vi "Score Particles2.vi"(6 "error in (no error)":errorcluster, 8 "Area Size Limit":i32=444, 9 "Particle Count Limit":i32=10, 11 "Image Refnum in":T1) -> (0 "error out":errorcluster, 2 "Scored Particle Info":T2(array[cluster]), 3 "Image Refnum out":T1)   [LabVIEW 2011]
doc: "Score the largest particles in the image to determine how well they match the target attributes. Specifically, calculate how rectangular a particle is, inspect its aspect ratio, and determine if it is hollow (having pixels on around the edges, but off in the large center)."
uses:
  <vilib>/vision/Image Controls.llb/IMAQ Image.ctl
  <vilib>/vision/NI_Vision_Development_Module.lvlib
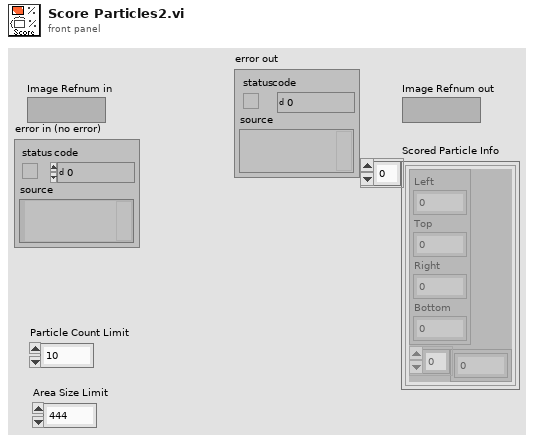
[diagram p1: front panel]
types:
  T1 = typedef "IMAQ Image.ctl" = refnum<image>
  T2 = cluster{cluster{"Left":dbl, "Top":dbl, "Right":dbl, "Bottom":dbl}, dbl[]}[]
  T3 = typedef "Particle Parameters" = i32
  T4 = typedef "Image Type" = u32
  T5 = cluster{"Left":dbl, "Top":dbl, "Right":dbl, "Bottom":dbl}
  T6 = cluster{cluster{"Left":dbl, "Top":dbl, "Right":dbl, "Bottom":dbl}, dbl[]}
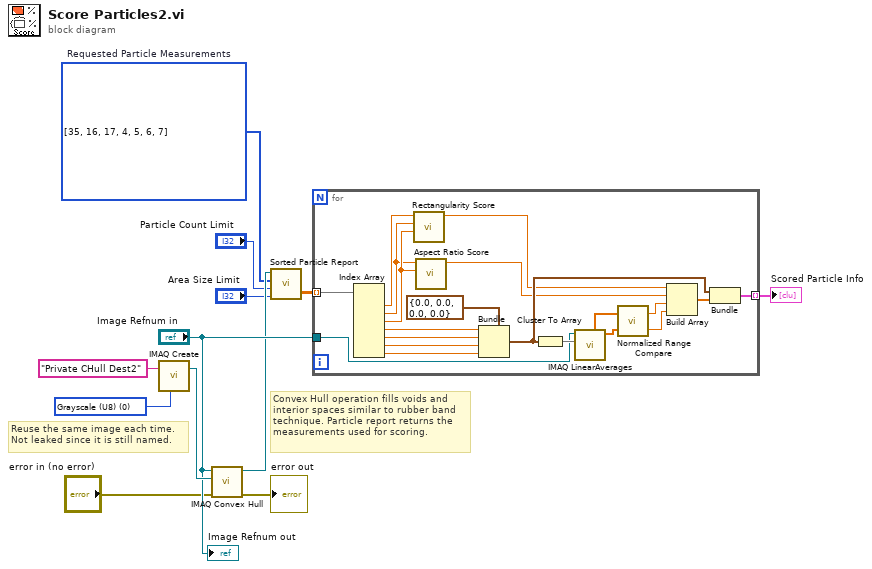
[diagram p0: block diagram]
diagram:
  w3 = T3[] [35, 16, 17, 4, 5, 6, 7] items=["Center of Mass X", "Center of Mass Y", "First Pixel X", "First Pixel Y", "Bounding Rect Left", "Bounding Rect Top", "Bounding Rect Right", "Bounding Rect Bottom", "Max Feret Diameter Start X", "Max Feret Diameter Start Y", "Max Feret Diameter End X", "Max Feret Diameter End Y", "Max Horiz. Segment Length Left", "Max Horiz. Segment Length Right", "Max Horiz. Segment Length Row", "-", "Bounding Rect Width", "Bounding Rect Height", "Bounding Rect Diagonal", "Perimeter", "Convex Hull Perimeter", "Holes' Perimeter", "Max Feret Diameter", "Equivalent Ellipse Major Axis", "Equivalent Ellipse Minor Axis", "Equivalent Ellipse Minor Axis (Feret)", "Equivalent Rect Long Side", "Equivalent Rect Short Side", "Equivalent Rect Diagonal", "Equivalent Rect Short Side (Feret)", "Average Horiz. Segment Length", "Average Vert. Segment Length", "Hydraulic Radius", "Waddel Disk Diameter", "-", "Area", "Holes' Area", "Particle & Holes' Area", "Convex Hull Area", "Image Area", "-", "Number of Holes", "Number of Horiz. Segments", "Number of Vert. Segments", "-", "Orientation", "Max Feret Diameter Orientation", "-", "% Area/Image Area", "% Area/(Particle & Holes' Area)", "Ratio of Equivalent Ellipse Axes", "Ratio of Equivalent Rect Sides", "-", "Elongation Factor", "Compactness Factor", "Heywood Circularity Factor", "Type Factor", "-", "Sum X", "Sum Y", "Sum XX", "Sum XY", "Sum YY", "Sum XXX", "Sum XXY", "Sum XYY", "Sum YYY", "-", "Moment of Inertia XX", "Moment of Inertia XY", "Moment of Inertia YY", "Moment of Inertia XXX", "Moment of Inertia XXY", "Moment of Inertia XYY", "Moment of Inertia YYY", "Norm. Moment of Inertia XX", "Norm. Moment of Inertia XY", "Norm. Moment of Inertia YY", "Norm. Moment of Inertia XXX", "Norm. Moment of Inertia XXY", "Norm. Moment of Inertia XYY", "Norm. Moment of Inertia YYY", "Hu Moment 1", "Hu Moment 2", "Hu Moment 3", "Hu Moment 4", "Hu Moment 5", "Hu Moment 6", "Hu Moment 7"]  # Requested Particle Measurements
  w9 = T4 0 items=["Grayscale (U8)", "Grayscale (I16)", "Grayscale (SGL)", "Complex (CSG)", "RGB (U32)", "HSL (U32)", "RGB (U64)", "Grayscale (U16)"] ("Image Type")
  # "Reuse the same image each time.\nNot leaked since it is still named."
  # "Convex Hull operation fills voids and\ninterior spaces similar to rubber band\ntechnique. Particle report returns the\nmeasurements used for scoring."
  n1 = call "IMAQ Create"("Image Name"="Private CHull Dest2", "Image Type"=w9) -> ("New Image"=w8:T1)  [unwired: 2 in, 2 out]
  n2 = call "IMAQ Convex Hull"("error in (no error)"="error in (no error)", "Image Dst"=w8, "Image Src"="Image Refnum in") -> ("error out"=→"error out":errorcluster, "Image Dst Out"=w6:T1)  [unwired: 1 in, 6 out]
  n3 = call "Sorted Particle Report.vi"("Area Size Limit"="Area Size Limit", "Particle Count Limit"="Particle Count Limit", "Pixel Measurements"=w3, "Image in"=w6) -> ("Sorted Data"=w11:dbl[][])  [unwired: 1 out]
  n4 = for {
    tunnel: [w30] -> w12 mode=indexing
    tunnel: "Image Refnum in" -> [w20]
    tunnel: w11 -> [w19] mode=indexing
    n5 = Index Array(array=w19) -> (element #1=w31:dbl, element #2=w13:dbl, element #3=w14:dbl, element #4=w15:dbl, element #5=w16:dbl, element #6=w17:dbl, element #7=w18:dbl)  [unwired: 7 in]
    n6 = call "Rectangularity Score.vi"("Height"=w14, "Width"=w13, "Area"=w31) -> ("Score"=w24:dbl)  [unwired: 8 in]
    n7 = call "Aspect Ratio Score.vi"("Height"=w14, "Width"=w13) -> ("Score"=w25:dbl)  [unwired: 9 in]
    n8 = Bundle(cluster=T5 {"Left"=0.0, "Top"=0.0, "Right"=0.0, "Bottom"=0.0}, "Left"=w15, "Top"=w16, "Right"=w17, "Bottom"=w18) -> (w29:T5)
    n9 = Cluster To Array(cluster=w29) -> (array=w21:dbl[])
    n10 = call "IMAQ LinearAverages"("Optional Rectangle"=w21, "Image Src"=w20) -> ("Y Axis Averages"=w23:sgl[], "X Axis Averages"=w22:sgl[])  [unwired: 2 in, 6 out]
    n11 = call "Normalized Range Compare.vi"("Y Averages"=w23, "X Averages"=w22) -> ("Y Score"=w27:dbl, "X Score"=w26:dbl)
    n12 = Build Array(w24, w25, w26, w27) -> (w28:dbl[])
    n13 = Bundle(w29, w28) -> (w30:T6)  [unwired: 1 in]
  }
  "Scored Particle Info" <- w12
  "Image Refnum out" <- "Image Refnum in"
